vi "Set Parameters.vi"(8 "error in (no error)":errorcluster, 10 "Parameters":refnum<class "PropertyObject.lvclass">, 11 "Execution in":refnum<class "Execution.lvclass">) -> (0 "error out":errorcluster, 3 "Execution out":refnum<class "Execution.lvclass">)   [LabVIEW 2020, in "TSnax.lvlib" / "Execution.lvclass"]
uses:
  Execution.lvclass
  Execution.lvclass/Execution.ctl
  PropertyObject/PropertyObject.lvclass
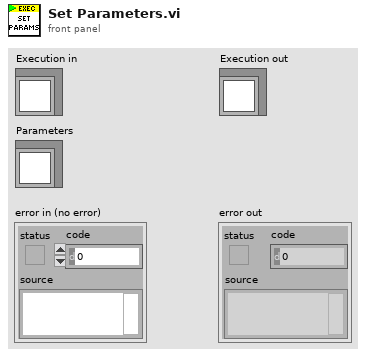
[diagram p1: front panel]
types:
  T1 = typedef "TSnax.lvlib/Execution.lvclass/Ref Data.ctl" = cluster{"Parameters":refnum<class "PropertyObject.lvclass">, "Client Sequence":refnum<class "SequenceFile.lvclass">, "Process Model":refnum<class "SequenceFile.lvclass">, "Entry Sequence":string, "Execution":refnum<k7>, "Report":refnum<class "Report.lvclass">, "Options":T2}
  T2 = typedef "TSnax.lvlib/Execution.lvclass/Execution Options.ctl" = cluster{"Use Default Model":bool, "Release Related Sessions":bool}
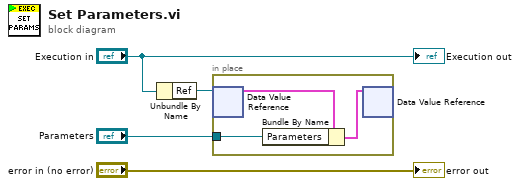
[diagram p0: block diagram]
diagram:
  n1 = Unbundle By Name("Execution in") -> ("Ref"=w3:refnum<data-value>)
  n2 = in-place {
    in-place-border: "Parameters" -> [w5]
    n3 = in-place-dvr #1(w3) -> (w7:T1)  [unwired: 1 out]
    n4 = Bundle By Name(cluster=w7, "Parameters"=w5) -> (w6:T1)
    n5 = in-place-dvr #1(w6) -> ()  [unwired: 2 out]
  }
  "error out" <- "error in (no error)"
  "Execution out" <- "Execution in"
